vi "ROI entry-bundle UI ctrl values.vi"(8 "error in (no error)":errorcluster, 10 "Input cluster":T1={"Imaging Protocol"=enum."AOL Z-Stack", "Number of POI"=0, "Number of Miniscans"=0, "Number of Trials"=0, "Number of Cycles "=0, "# Averaged Frames"=0, "Laser power (%)"=0, "Pockels"=0.0, "Acquisition Length (sec)"=0.0, "Fill time (us)"=0.0, "POI Dwell time (us)"=0.0, "Miniscan Dwell time per pixel (us)"=0.0, "PMT 1"=0.0, "PMT 2"=0.0, "Back Apperture"=0.0, "Frame Size"=0, "Center Frequency"=0.0, "Field of View"=0.0, "DwellTime (us)"=0.0, "Wavelength (nm)"=0.0, "Zoom"=0.0, "AOL Z"=0.0, "AOL Mode"=enum."Raster", "GridXY"=0.0, "GridZ"=0.0, "TriggerPeriod (sec)"=0.0, "Number of Pixels in Miniscan"=0, "Experiment folder path"=path "", "X centre"=0.0, "Y centre"=0.0, "Angle (degrees)"=0.0, "Plane Mode"=0, "Threshold"=[], "Regenerate Chirps"=FALSE, "Rectangle ROI length (pixels)"=0, "Rectangle ROI height (pixels)"=0, "AOD fill"=0, "Samples Wait after Trigger"=0, "StartUp Delay"=0, "Slip Cycle"=163840, "Add Cycle"=FALSE} {"Plane Mode" items=["XY Plane"]; "Frame Size" items=["100X100"=100, "128X128"=128, "200X200"=200, "256X256"=256, "512X512"=512, "1024x1024"=1024, "2048x2048"=2048]; "Back Apperture" format="%#.6g"; "Pockels" format="%#.6g"; "PMT 2" format="%#.6g"; "PMT 1" format="%#.6g"; "Angle (degrees)" format="%#.6g"; "POI Dwell time (us)" format="%#.6g"}) -> (0 "Error Out":errorcluster, 2 "Output cluster":T1={"Imaging Protocol"=enum."Live Imaging", "Number of POI"=0, "Number of Miniscans"=0, "Number of Trials"=0, "Number of Cycles "=0, "# Averaged Frames"=0, "Laser power (%)"=0, "Pockels"=0.0, "Acquisition Length (sec)"=0.0, "Fill time (us)"=0.0, "POI Dwell time (us)"=0.0, "Miniscan Dwell time per pixel (us)"=0.0, "PMT 1"=0.0, "PMT 2"=0.0, "Back Apperture"=0.0, "Frame Size"=200, "Center Frequency"=0.0, "Field of View"=0.0, "DwellTime (us)"=0.0, "Wavelength (nm)"=0.0, "Zoom"=0.0, "AOL Z"=0.0, "AOL Mode"=enum."Raster", "GridXY"=0.0, "GridZ"=0.0, "TriggerPeriod (sec)"=0.0, "Number of Pixels in Miniscan"=0, "Experiment folder path"=path "", "X centre"=0.0, "Y centre"=0.0, "Angle (degrees)"=0.0, "Plane Mode"=0, "Threshold"=[], "Regenerate Chirps"=FALSE, "Rectangle ROI length (pixels)"=0, "Rectangle ROI height (pixels)"=0, "AOD fill"=0, "Samples Wait after Trigger"=0, "StartUp Delay"=0, "Slip Cycle"=163840, "Add Cycle"=FALSE} {"Plane Mode" items=["XY Plane"]; "Frame Size" items=["100X100"=100, "128X128"=128, "200X200"=200, "256X256"=256, "512X512"=512, "1024x1024"=1024, "2048x2048"=2048]; "Back Apperture" format="%#.6g"; "Pockels" format="%#.6g"; "PMT 2" format="%#.6g"; "PMT 1" format="%#.6g"; "Angle (degrees)" format="%#.6g"; "POI Dwell time (us)" format="%#.6g"})   [LabVIEW 2013]
uses:
  Typedefs/Controls/AOL_Globals.ctl
  Typedefs/Imaging Protocols enum.ctl
  Typedefs/Frame Size.ctl
  Typedefs/AOL modes.ctl
  Typedefs/Plane Mode.ctl
  ROI Entry screen/Globals/gl_ROI Entry UI globals.vi
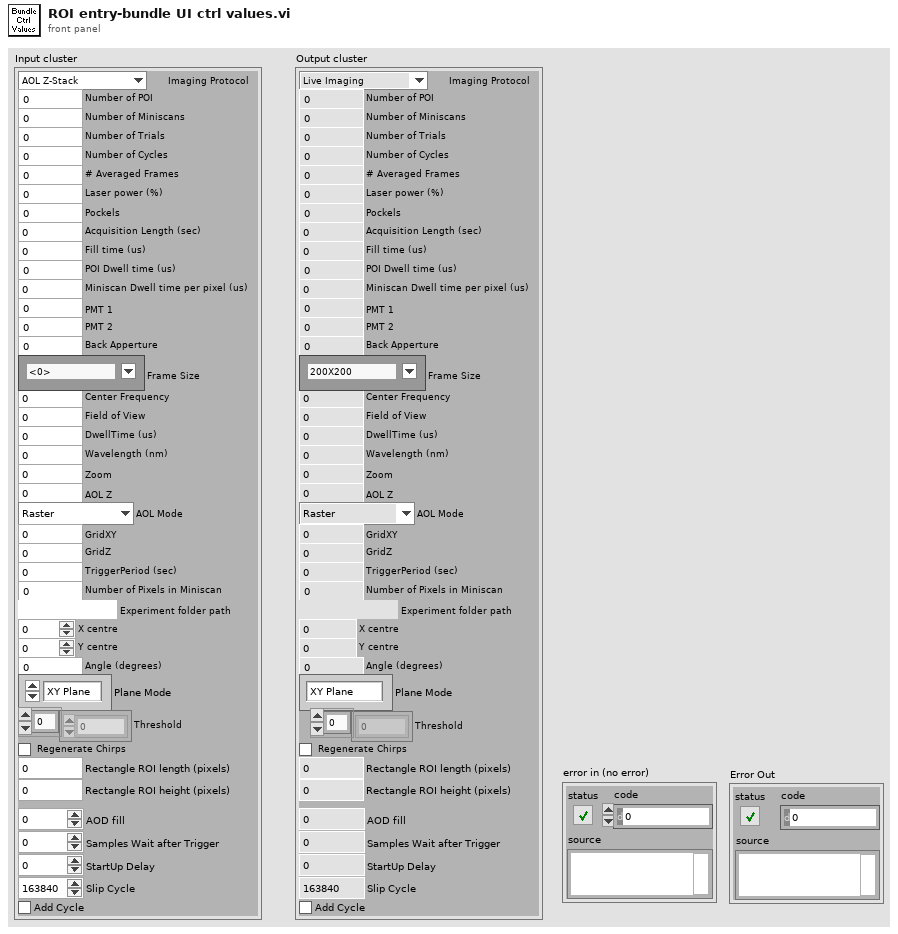
[diagram p1: front panel]
types:
  T1 = typedef "AOL_Globals.ctl" = cluster{"Imaging Protocol":T2, "Number of POI":u16, "Number of Miniscans":u16, "Number of Trials":u16, "Number of Cycles ":u64, "# Averaged Frames":u16, "Laser power (%)":u8, "Pockels":dbl, "Acquisition Length (sec)":dbl, "Fill time (us)":dbl, "POI Dwell time (us)":dbl, "Miniscan Dwell time per pixel (us)":dbl, "PMT 1":dbl, "PMT 2":dbl, "Back Apperture":dbl, "Frame Size":T3, "Center Frequency":dbl, "Field of View":dbl, "DwellTime (us)":dbl, "Wavelength (nm)":dbl, "Zoom":dbl, "AOL Z":dbl, "AOL Mode":T4, "GridXY":dbl, "GridZ":dbl, "TriggerPeriod (sec)":dbl, "Number of Pixels in Miniscan":u16, "Experiment folder path":path, "X centre":dbl, "Y centre":dbl, "Angle (degrees)":dbl, "Plane Mode":T5, "Threshold":u16[], "Regenerate Chirps":bool, "Rectangle ROI length (pixels)":u16, "Rectangle ROI height (pixels)":u16, "AOD fill":u16, "Samples Wait after Trigger":u16, "StartUp Delay":i32, "Slip Cycle":u32, "Add Cycle":bool}
  T2 = typedef "Imaging Protocols enum.ctl" = enum16{"AOL Z-Stack", "Motor Z Stack", "Functional Acquisition", "Single Plane Acquisition", "Volume Acquisition", "Live Imaging", "Live Plane Imaging", "Live Volume Imaging"}
  T3 = typedef "Frame Size.ctl" = u16
  T4 = typedef "AOL modes.ctl" = enum16{"Raster", "Structural", "Pointing", "Mini Scan", "Alignment"}
  T5 = typedef "Plane Mode.ctl" = u16
  T6 = typedef "ROI entry screen ctrl refs cluster.ctl" = cluster{"Done button":refnum<vi>, "Imaging button":refnum<vi>, "Acquisition button":refnum<vi>, "POI dwell time (us)":refnum<vi>, "Scan dwell time per pixel (us)":refnum<vi>, "# of planes":refnum<vi>, "Zoom":refnum<vi>, "Equal size":refnum<vi>, "Channel":refnum<vi>, "Image Display":refnum<vi>, "Z-Plane Selector":refnum<vi>, "Number of lines left":refnum<vi>, "Z-stack folder path":refnum<vi>, "POI Density":refnum<vi>, "Arb Plane Entry":refnum<vi>, "Whole plane":refnum<vi>, "Clear Last":refnum<vi>, "Clear All":refnum<vi>, "Trial Length (sec)":refnum<vi>, "Palette Type":refnum<vi>, "Intensity slider":refnum<vi>, "# POI":refnum<vi>, "Max Z Proj":refnum<vi>, "Zplane ind":refnum<vi>, "Wavelength (nm)":refnum<vi>, "Number of Trials":refnum<vi>, "Funct stim.trig.enable":refnum<vi>, "Funct stim.trig.delay (s)":refnum<vi>, "Line Mode":refnum<vi>, "Step size (µm)":refnum<vi>, "ROI move mode":refnum<vi>, "Cool-down time (s)":refnum<vi>, "Enable cool-down time":refnum<vi>, "Motor Z ind. (um)":refnum<vi>, "AOL Z ind. (um)":refnum<vi>}
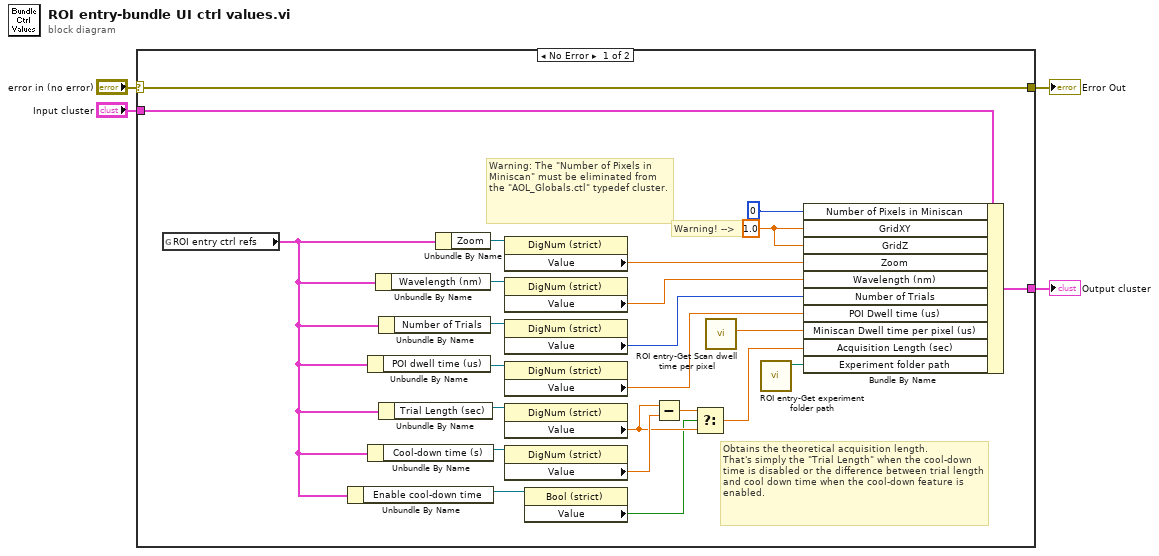
[diagram p0: block diagram]
diagram:
  n1 = case shown="No Error" "error in (no error)" {
    selector: "error in (no error)" -> [w15 w30]
    tunnel: [w18 w29] -> w4
    tunnel: "Input cluster" -> [w17 w29]
    tunnel: [w15 w30] -> w1
    frame No Error {
      w19 = 1.0 ("GridXY")
      # "Obtains the theoretical acquisition length.\nThat's simply the \"Trial Length\" when the cool-down time is disabled or the difference between trial length and cool down time when the cool-down feature is enabled."
      # "Warning: The \"Number of Pixels in Miniscan\" must be eliminated from the \"AOL_Globals.ctl\" typedef cluster."
      # "Warning! -->"
      n2 = global read "gl_ROI Entry UI globals.vi" "ROI entry ctrl refs"() -> (w9:T6)
      n3 = Unbundle By Name(w9) -> ("Enable cool-down time"=w10:refnum<vi>)
      n4 = Unbundle By Name(w9) -> ("POI dwell time (us)"=w25:refnum<vi>)
      n5 = Unbundle By Name(w9) -> ("Cool-down time (s)"=w12:refnum<vi>)
      n6 = Unbundle By Name(w9) -> ("Wavelength (nm)"=w27:refnum<vi>)
      n7 = Unbundle By Name(w9) -> ("Number of Trials"=w26:refnum<vi>)
      n8 = Unbundle By Name(w9) -> ("Trial Length (sec)"=w24:refnum<vi>)
      n9 = Unbundle By Name(w9) -> ("Zoom"=w28:refnum<vi>)
      n10 = property on="Property Node" class="DigNum (strict)"(reference=w28) -> ("Value"=w23:dbl)  [unwired: 1 in, 2 out]
      n11 = property on="Property Node" class="DigNum (strict)"(reference=w27) -> ("Value"=w22:dbl)  [unwired: 1 in, 2 out]
      n12 = property on="Property Node" class="DigNum (strict)"(reference=w26) -> ("Value"=w21:u16)  [unwired: 1 in, 2 out]
      n13 = property on="Property Node" class="DigNum (strict)"(reference=w25) -> ("Value"=w20:dbl)  [unwired: 1 in, 2 out]
      n14 = property on="Property Node" class="DigNum (strict)"(reference=w24) -> ("Value"=w8:dbl)  [unwired: 1 in, 2 out]
      n15 = property on="Property Node" class="DigNum (strict)"(reference=w12) -> ("Value"=w11:dbl)  [unwired: 1 in, 2 out]
      n16 = property on="Property Node" class="Bool (strict)"(reference=w10) -> ("Value"=w7:bool)  [unwired: 1 in, 2 out]
      n17 = Subtract(x=w8, y=w11) -> (x-y=w6:dbl)
      n18 = Select(t=w6, s=w7, f=w8) -> (s? t:f=w5:dbl)
      n19 = call "ROI entry-Get Scan dwell time per pixel.vi"() -> ("Scan dwell time per pixel (us)"=w13:dbl)  [unwired: 10 in, 1 out]
      n20 = call "ROI entry-Get experiment folder path.vi"() -> ("Experiment folder path"=w14:path)  [unwired: 10 in, 1 out]
      n21 = Bundle By Name(cluster=w17, "Number of Pixels in Miniscan"=u16 0, "GridXY"=w19, "GridZ"=w19, "Zoom"=w23, "Wavelength (nm)"=w22, "Number of Trials"=w21, "POI Dwell time (us)"=w20, "Miniscan Dwell time per pixel (us)"=w13, "Acquisition Length (sec)"=w5, "Experiment folder path"=w14) -> (w18:T1)
    }
    frame Error {
    }
  }
  "Output cluster" <- w4
  "Error Out" <- w1
